vi "E _1629 measurement.vi"(8 "error in (no error)":errorcluster, 9 "Calibrated Image":T2, 10 "1629 E Input Cluster":T8={"Meas ROI-2 After Transformation"={"Global Rectangle"=[131, 293, 235, 470], "Contours"=[{"ID"=enum."External", "Type"=12, "Coordinates"=[133, 294, 233, 469, -359104]}]}, "Meas ROI -1 After Transformation"={"Global Rectangle"=[646, 271, 718, 353], "Contours"=[{"ID"=enum."External", "Type"=12, "Coordinates"=[647, 272, 717, 352, -359104]}]}, "Meas ROI-2 Search Direction"=0, "Meas ROI-1 Search Direction"=0, "Meas ROI-2 Edge Options"={"Edge Polarity"=2, "Kernel Size"=5, "Width"=5, "Minimum Edge Strength"=50.0, "Interpolation Type"=enum."Zero Order", "Data Processing Method"=enum."Average"}, "Meas ROI-1 Edge Options"={"Edge Polarity"=2, "Kernel Size"=5, "Width"=5, "Minimum Edge Strength"=50.0, "Interpolation Type"=enum."Zero Order", "Data Processing Method"=enum."Average"}, "1629 E Ref Straight Edges"=[{"Point1 (Pixels)"={"X"=381.67548, "Y"=327.23843}, "Point2 (Pixels)"={"X"=493.65692, "Y"=325.05707}, "Point1 (Real-World)"={"X"=381.67548, "Y"=327.23843}, "Point2 (Real-World)"={"X"=493.65692, "Y"=325.05707}, "Angle (Pixel)"=0.19930062632701423, "Angle (Real-World)"=0.19930062632701423, "Score"=427.45098039215685, "Straightness"=0.1545564593431227, "Average SNR (db)"=23.448024809056935, "Calibration Valid"=TRUE}], "Meas ROI-1 Line Options"={"Number of Lines"=1, "Type"=enum."Best Edge Projection", "Min. Score"=10.0, "Max. Score"=1000.0, "Orientation"=0.0, "Angle Range"=10.0, "Angle Tolerance"=1.0, "Step Size"=3, "Min. SNR (db)"=0.0, "Min. Points (%)"=25.0, "Hough Iterations"=5}, "Meas ROI-2 Line Options"={"Number of Lines"=1, "Type"=enum."Best Edge Rake", "Min. Score"=10.0, "Max. Score"=1000.0, "Orientation"=0.0, "Angle Range"=30.0, "Angle Tolerance"=1.0, "Step Size"=3, "Min. SNR (db)"=0.0, "Min. Points (%)"=25.0, "Hough Iterations"=5}} {"Meas ROI-2 Line Options"."Min. Points (%)" min=0.0 max=100.0; "Meas ROI-2 Line Options"."Min. SNR (db)" min=0.0; "Meas ROI-2 Line Options"."Max. Score" min=0.0 max=1024.0; "Meas ROI-2 Line Options"."Min. Score" min=0.0 max=1024.0 step=1.0; "Meas ROI-1 Line Options"."Min. Points (%)" min=0.0 max=100.0; "Meas ROI-1 Line Options"."Min. SNR (db)" min=0.0; "Meas ROI-1 Line Options"."Max. Score" min=0.0 max=1024.0; "Meas ROI-1 Line Options"."Min. Score" min=0.0 max=1024.0 step=1.0; "1629 E Ref Straight Edges"."Point2 (Real-World)"."Y" format="%.2f"; "1629 E Ref Straight Edges"."Point2 (Real-World)"."X" format="%.2f"; "1629 E Ref Straight Edges"."Point1 (Real-World)"."Y" format="%.2f"; "1629 E Ref Straight Edges"."Point1 (Real-World)"."X" format="%.2f"; "1629 E Ref Straight Edges"."Point2 (Pixels)"."Y" format="%.2f"; "1629 E Ref Straight Edges"."Point2 (Pixels)"."X" format="%.2f"; "1629 E Ref Straight Edges"."Point1 (Pixels)"."Y" format="%.2f"; "1629 E Ref Straight Edges"."Point1 (Pixels)"."X" format="%.2f"; "Meas ROI-1 Edge Options"."Edge Polarity" items=["All Edges", "Rising Edges", "Falling Edges"]; "Meas ROI-1 Edge Options"."Minimum Edge Strength" format="%.2f"; "Meas ROI-1 Edge Options"."Width" step=2; "Meas ROI-1 Edge Options"."Kernel Size" step=2; "Meas ROI-2 Edge Options"."Edge Polarity" items=["All Edges", "Rising Edges", "Falling Edges"]; "Meas ROI-2 Edge Options"."Minimum Edge Strength" format="%.2f"; "Meas ROI-2 Edge Options"."Width" step=2; "Meas ROI-2 Edge Options"."Kernel Size" step=2; "Meas ROI-1 Search Direction" items=["Left to Right", "Right to Left", "Top to Bottom", "Bottom to Top"]; "Meas ROI-2 Search Direction" items=["Left to Right", "Right to Left", "Top to Bottom", "Bottom to Top"]; "Meas ROI -1 After Transformation"."Contours"."Type" items=["No Selection", "Point", "Line", "Rectangle", "Oval", "Polygon", "Freehand Region", "Annulus", "Unused2", "Unused3", "Broken Line", "Freehand Line", "Rotated Rectangle"]; "Meas ROI-2 After Transformation"."Contours"."Type" items=["No Selection", "Point", "Line", "Rectangle", "Oval", "Polygon", "Freehand Region", "Annulus", "Unused2", "Unused3", "Broken Line", "Freehand Line", "Rotated Rectangle"]}, 11 "Input Image":T2) -> (0 "error out":errorcluster, 2 "output cluster":T1, 3 "Result Image":T2(plugin-control))   [LabVIEW 2019, in "Algorithm.lvclass"]
doc: "Description:\nThis VI Required Input image, Calibrated image and input Cluster. The input Cluster Contains two ROIs, Two Search Directions , Two Edge options. The two ROIs and Search directions are used to find the straight line. From these lines, find middle poins for each line.\nThen seprately find perpendicular intersection points from middle points of straight lines and Ref Straight Edges. Finally Measure the distance using these intersection points."
uses:
  FrameworkOverrides/Algorithm.lvclass
  <vilib>/vision/NI_Vision_Development_Module.lvlib
  <vilib>/vision/Image Controls.llb/IMAQ Image.ctl
  <vilib>/vision/Measure.llb/Edge Polarity.ctl
  <vilib>/vision/Measure.llb/Edge Options.ctl
  <vilib>/vision/Measure.llb/Straight Edge Process.ctl
  <vilib>/vision/Measure.llb/Straight Edge Options.ctl
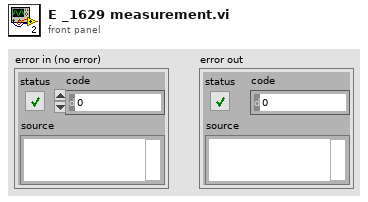
[diagram p1: front panel]
types:
  T1 = cluster{"Points for Overlay":cluster{"Point 2":cluster{"X":sgl, "Y":sgl}, "Point 2":cluster{"X":sgl, "Y":sgl}}, "E Measurement":sgl}
  T2 = typedef "IMAQ Image.ctl" = refnum<image>
  T3 = typedef "ROI Descriptor" = cluster{"Global Rectangle":i32[], "Contours":cluster{"ID":enum32{"External", "Internal"}, "Type":u32, "Coordinates":i32[]}[]}
  T4 = typedef "Edge Options.ctl" = cluster{"Edge Polarity":T5, "Kernel Size":u32, "Width":u32, "Minimum Edge Strength":sgl, "Interpolation Type":enum32{"Zero Order", "Bilinear", "Quadratic", "Cubic", "Bilinear Fixed"}, "Data Processing Method":enum32{"Average", "Median"}}
  T5 = typedef "Edge Polarity.ctl" = u32
  T6 = typedef "Straight Edge Options.ctl" = cluster{"Number of Lines":i32, "Type":T7, "Min. Score":dbl, "Max. Score":dbl, "Orientation":dbl, "Angle Range":dbl, "Angle Tolerance":dbl, "Step Size":u32, "Min. SNR (db)":dbl, "Min. Points (%)":dbl, "Hough Iterations":i32}
  T7 = typedef "Straight Edge Process.ctl" = enum32{"First Edge Rake", "Best Edge Rake", "Hough Edge Rake", "First Edge Projection", "Best Edge Projection"}
  T8 = cluster{"Meas ROI-2 After Transformation":T3, "Meas ROI -1 After Transformation":T3, "Meas ROI-2 Search Direction":u32, "Meas ROI-1 Search Direction":u32, "Meas ROI-2 Edge Options":T4, "Meas ROI-1 Edge Options":T4, "1629 E Ref Straight Edges":cluster{"Point1 (Pixels)":cluster{"X":sgl, "Y":sgl}, "Point2 (Pixels)":cluster{"X":sgl, "Y":sgl}, "Point1 (Real-World)":cluster{"X":sgl, "Y":sgl}, "Point2 (Real-World)":cluster{"X":sgl, "Y":sgl}, "Angle (Pixel)":dbl, "Angle (Real-World)":dbl, "Score":dbl, "Straightness":dbl, "Average SNR (db)":dbl, "Calibration Valid":bool}[], "Meas ROI-1 Line Options":T6, "Meas ROI-2 Line Options":T6}
  T9 = cluster{"Point 1":cluster{"X":sgl, "Y":sgl}, "Point 2":cluster{"X":sgl, "Y":sgl}}
  T10 = cluster{"Point1 (Pixels)":cluster{"X":sgl, "Y":sgl}, "Point2 (Pixels)":cluster{"X":sgl, "Y":sgl}, "Point1 (Real-World)":cluster{"X":sgl, "Y":sgl}, "Point2 (Real-World)":cluster{"X":sgl, "Y":sgl}, "Angle (Pixel)":dbl, "Angle (Real-World)":dbl, "Score":dbl, "Straightness":dbl, "Average SNR (db)":dbl, "Calibration Valid":bool}[]
  T11 = cluster{"Point1 (Pixels)":cluster{"X":sgl, "Y":sgl}, "Point2 (Pixels)":cluster{"X":sgl, "Y":sgl}, "Point1 (Real-World)":cluster{"X":sgl, "Y":sgl}, "Point2 (Real-World)":cluster{"X":sgl, "Y":sgl}, "Angle (Pixel)":dbl, "Angle (Real-World)":dbl, "Score":dbl, "Straightness":dbl, "Average SNR (db)":dbl, "Calibration Valid":bool}
  T12 = cluster{"Point 2":cluster{"X":sgl, "Y":sgl}, "Point 2":cluster{"X":sgl, "Y":sgl}}
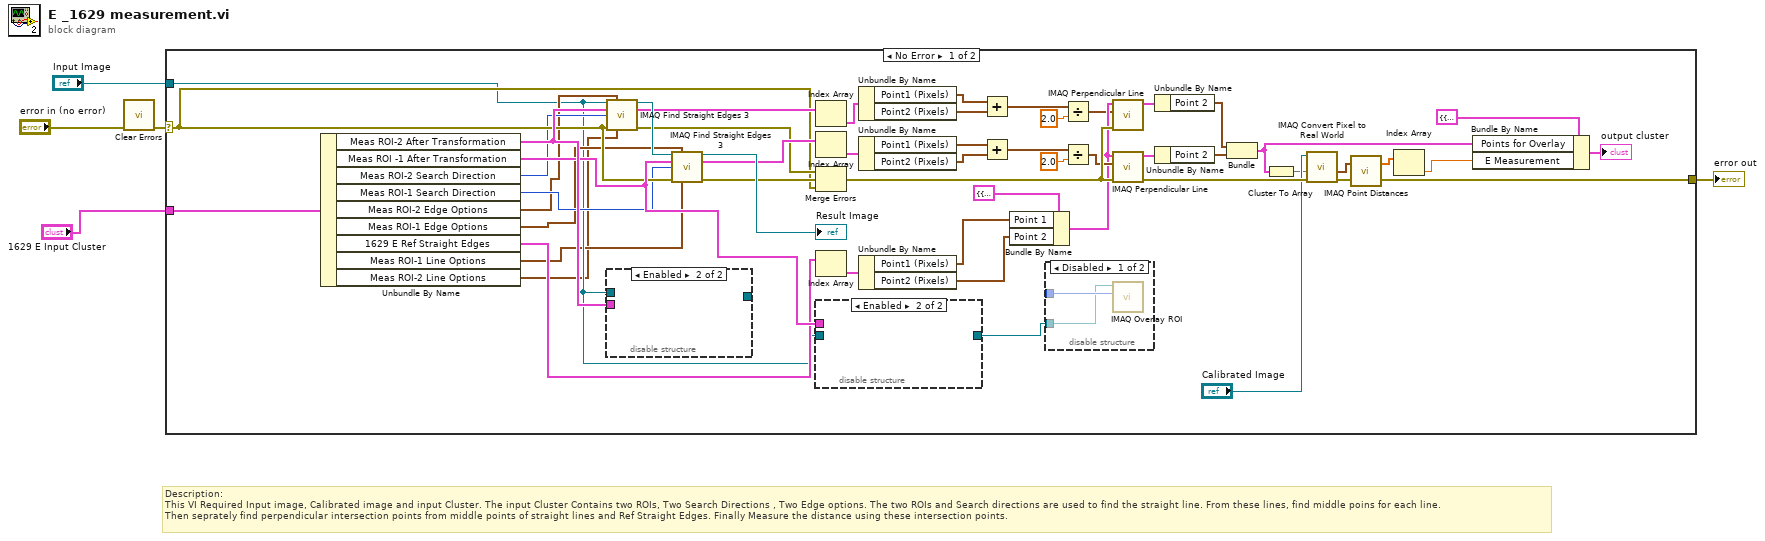
[diagram p0: block diagram]
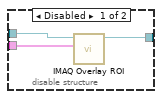
[diagram p2: hidden frame]
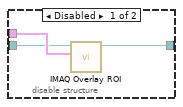
[diagram p4: hidden frame]
diagram:
  # "Description:\nThis VI Required Input image, Calibrated image and input Cluster. The input Cluster Contains two ROIs, Two Search Directions , Two Edge options. The two ROIs and Search directions are used to find the straight line. From these lines, find middle poins for each line.\nThen seprately find perpendicular intersection points from middle points of straight lines and Ref Straight Edges. Finally Measure the distance using these intersection points."
  n1 = call <vilib>:"Clear Errors.vi"("error in (no error)"="error in (no error)") -> ("error out"=w4:errorcluster)  [unwired: 5 in, 1 out]
  n2 = case shown="No Error" w4 {
    selector: w4 -> [w17 w66]
    tunnel: [w18 w66] -> w3
    tunnel: "1629 E Input Cluster" -> [w16 _]
    tunnel: "Input Image" -> [w8 _]
    frame No Error {
      n3 = Unbundle By Name(w16) -> ("Meas ROI-2 After Transformation"=w22:T3, "Meas ROI -1 After Transformation"=w21:T3, "Meas ROI-2 Search Direction"=w13:u32, "Meas ROI-1 Search Direction"=w12:u32, "Meas ROI-2 Edge Options"=w11:T4, "Meas ROI-1 Edge Options"=w10:T4, "1629 E Ref Straight Edges"=w9:T10, "Meas ROI-1 Line Options"=w7:T6, "Meas ROI-2 Line Options"=w6:T6)
      n4 = call "IMAQ Find Straight Edges 3"("Image"=w8, "Edge Options"=w11, "ROI Descriptor"=w22, "Search Direction"=w13, "error in (no error)"=w17, "Line Options"=w6) -> ("Image (duplicate)"=w37:T2, "Straight Edges"=w35:T10, "error out"=w34:errorcluster)  [unwired: 5 in, 2 out]
      n5 = disable-structure shown="Enabled" {
        disable-tunnel: w22 -> [w60 _]
        disable-tunnel: w8 -> [w59 _]
        disable-tunnel: [w58 _] -> _
        frame Disabled {
          n6 = call "IMAQ Overlay ROI"("ROI Descriptor"=w60, "Image"=w59) -> ("Image Out"=w58:T2)  [unwired: 8 in, 1 out]
        }
        frame Enabled {
        }
      }
      n7 = call "IMAQ Find Straight Edges 3"("Image"=w37, "Edge Options"=w10, "ROI Descriptor"=w21, "Search Direction"=w12, "error in (no error)"=w17, "Line Options"=w7) -> ("Image (duplicate)"=→"Result Image":T2, "Straight Edges"=w39:T10, "error out"=w33:errorcluster)  [unwired: 5 in, 2 out]
      n8 = Index Array(array=w35) -> (element=w36:T11)  [unwired: 1 in]
      n9 = Index Array(array=w39) -> (element=w38:T11)  [unwired: 1 in]
      n10 = Merge Errors(w34, w33, w17) -> (w54:errorcluster)
      n11 = Index Array(array=w9) -> (element=w41:T11)  [unwired: 1 in]
      n12 = disable-structure shown="Enabled" {
        disable-tunnel: w21 -> [w65 _]
        disable-tunnel: w8 -> [w64 _]
        disable-tunnel: [w63 _] -> w20
        frame Disabled {
          n13 = call "IMAQ Overlay ROI"("ROI Descriptor"=w65, "Image"=w64) -> ("Image Out"=w63:T2)  [unwired: 8 in, 1 out]
        }
        frame Enabled {
        }
      }
      n14 = Unbundle By Name(w36) -> ("Point1 (Pixels)"=w42:cluster{"X":sgl, "Y":sgl}, "Point2 (Pixels)"=w43:cluster{"X":sgl, "Y":sgl})
      n15 = Unbundle By Name(w38) -> ("Point1 (Pixels)"=w48:cluster{"X":sgl, "Y":sgl}, "Point2 (Pixels)"=w49:cluster{"X":sgl, "Y":sgl})
      n16 = Unbundle By Name(w41) -> ("Point1 (Pixels)"=w15:cluster{"X":sgl, "Y":sgl}, "Point2 (Pixels)"=w14:cluster{"X":sgl, "Y":sgl})
      n17 = Add(x=w42, y=w43) -> (x+y=w45:cluster{"X":sgl, "Y":sgl})
      n18 = Add(x=w48, y=w49) -> (x+y=w46:cluster{"X":sgl, "Y":sgl})
      n19 = Bundle By Name(cluster=T9 {"Point 1"={"X"=0.0, "Y"=0.0}, "Point 2"={"X"=0.0, "Y"=0.0}} ("Line"), "Point 1"=w15, "Point 2"=w14) -> (w52:T9)
      n20 = disable-structure shown="Disabled" {
        disable-tunnel: _ -> [w62 _]
        disable-tunnel: w20 -> [w61 _]
        frame Disabled {
          n21 = call "IMAQ Overlay ROI"("ROI Descriptor"=w62, "Image"=w61) -> ()  [unwired: 8 in, 2 out]
        }
        frame Enabled {
        }
      }
      n22 = Divide(x=w45, y=2.0) -> (x/y=w51:cluster{"X":dbl, "Y":dbl})
      n23 = Divide(x=w46, y=2.0) -> (x/y=w53:cluster{"X":dbl, "Y":dbl})
      n24 = call "IMAQ Perpendicular Line"("error in (no error)"=w54, "Point"=w51, "Line"=w52) -> ("Perpendicular Line"=w55:T9)  [unwired: 6 in, 2 out]
      n25 = call "IMAQ Perpendicular Line"("error in (no error)"=w54, "Point"=w53, "Line"=w52) -> ("error out"=w57:errorcluster, "Perpendicular Line"=w56:T9)  [unwired: 6 in, 1 out]
      n26 = Unbundle By Name(w55) -> ("Point 2"=w28:cluster{"X":sgl, "Y":sgl})
      n27 = Unbundle By Name(w56) -> ("Point 2"=w27:cluster{"X":sgl, "Y":sgl})
      n28 = Bundle("Point 2"=w28, "Point 2"=w27) -> (w23:T12)  [unwired: 1 in]
      n29 = Cluster To Array(cluster=w23) -> (array=w24:cluster{"X":sgl, "Y":sgl}[])
      n30 = call "IMAQ Convert Pixel to Real World"("error in (no error)"=w57, "Array of Pixel Coordinates"=w24, "Calibrated Image"="Calibrated Image") -> ("error out"=w30:errorcluster, "Array of Real World Coordinates"=w31:cluster{"X":sgl, "Y":sgl}[])  [unwired: 3 in, 4 out]
      n31 = call "IMAQ Point Distances"("Points"=w31, "error in (no error)"=w30) -> ("Distances"=w29:sgl[], "error out"=w18:errorcluster)  [unwired: 3 in]
      n32 = Index Array(array=w29) -> (element=w25:sgl)  [unwired: 1 in]
      n33 = Bundle By Name(cluster=T1 {"Points for Overlay"={"Point 2"={"X"=0.0, "Y"=0.0}, "Point 2"={"X"=0.0, "Y"=0.0}}, "E Measurement"=0.0}, "Points for Overlay"=w23, "E Measurement"=w25) -> (→"output cluster":T1)
    }
    frame Error {
    }
  }
  "error out" <- w3
